vi "PRN Read.vi"(8 "error in (no error)":errorcluster, 11 "prn":string="Barcode_Prn data") -> (0 "error out":errorcluster, 2 "Read Prn":string)   [LabVIEW 2015]
panel:
  # "C:\\Users\\AJAY\\Desktop\\TSC Barcode\\data\\Barcode\\Barcode-prn1.prn"
  # "Error code"
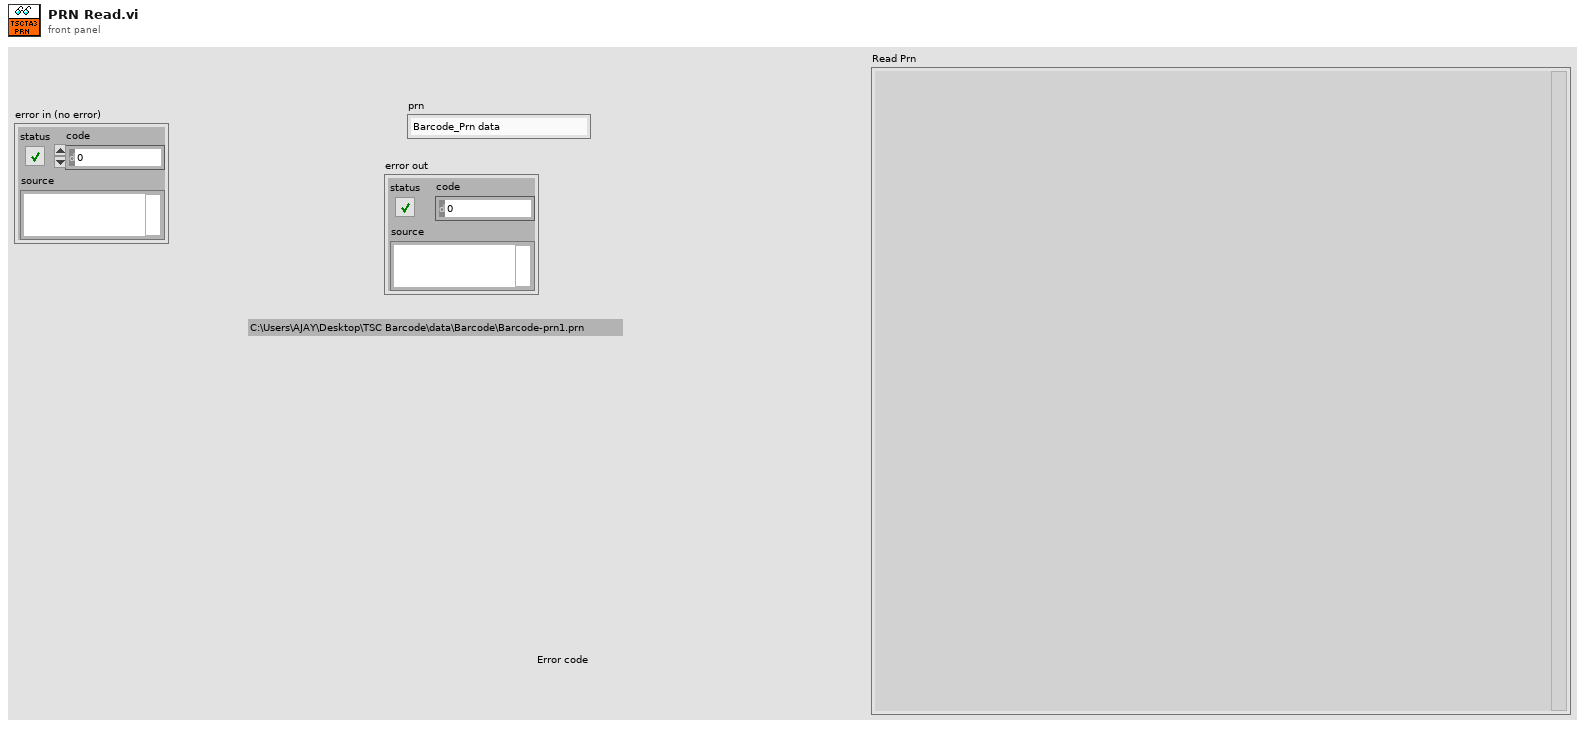
[diagram p1: front panel]
types:
  T1 = enum16{"open", "replace", "create", "open or create", "replace or create", "replace or create with confirmation"}
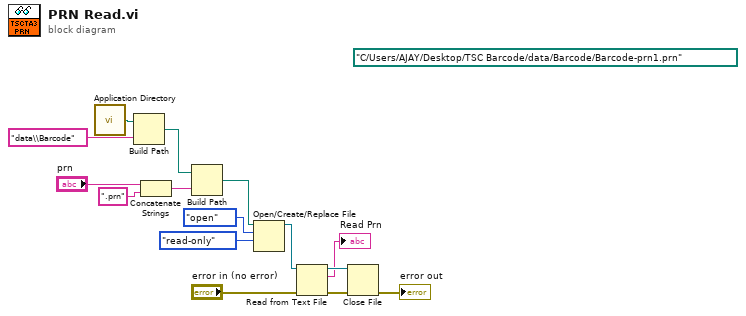
[diagram p0: block diagram]
diagram:
  (unwired) path "C:/Users/AJAY/Desktop/TSC Barcode/data/Barcode/Barcode-prn1.prn" ("file path (dialog if empty)")
  n1 = call <vilib>:"Application Directory.vi"() -> ("Application Directory"=w2:path)
  n2 = Build Path(base path=w2, name or relative path="data\\Barcode" ("string")) -> (appended path=w1:path)
  n3 = Concatenate Strings("prn", ".prn" ("string")) -> (w7:string)
  n4 = Build Path(base path=w1, name or relative path=w7) -> (appended path=w3:path)
  n5 = Open/Create/Replace File(file path (use dialog)=w3, operation (0:open)=T1."open", access (0:read/write)=enum16{"read/write", "read-only", "write-only"}."read-only") -> (refnum out=w12:refnum<file>)  [unwired: 3 in, 2 out]
  n6 = Read from Text File(file (use dialog)=w12, error in="error in (no error)") -> (refnum out=w13:refnum<file>, text=→"Read Prn":string, error out=w14:errorcluster)  [unwired: 2 in, 1 out]
  n7 = Close File(refnum=w13, error in=w14) -> (error out=→"error out":errorcluster)  [unwired: 1 out]
